vi "add_data_path_multiple.vi"(8 "error in (no error)":errorcluster, 11 "path_to_add []":path[](array[path])) -> (0 "error out":errorcluster)   [LabVIEW 2015, in "lv-bin.lvlib" / "v1.lvlib"]
uses:
  v1.lvlib
  private/_controls/fg_command.ctl
  lv-bin.lvlib
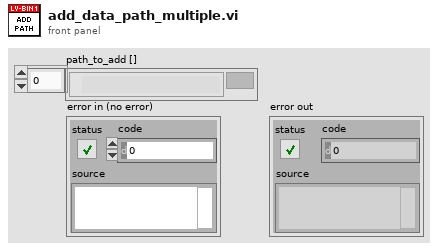
[diagram p1: front panel]
types:
  T1 = typedef "lv-bin.lvlib/fg_command.ctl" = enum16{"<fg_command>", "initialize", "read", "write", "shutdown", "<null>"}
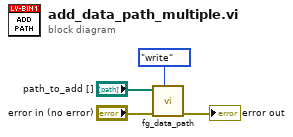
[diagram p0: block diagram]
diagram:
  n1 = call "fg_data_path.vi"("fg_command"=fg_command."write", "error in (no error)"="error in (no error)", "path [] in"="path_to_add []") -> ("error out"=→"error out":errorcluster)  [unwired: 7 in, 1 out]
